vi "Make_SQL_for_basic_param.vi"(6 "Material Type":string, 8 "Porosity, %":string, 9 "Hardness HV, kg/mm2":string, 10 "Thickness, um":string, 11 "Breakdown DC voltage, V":string) -> (3 "result string":string)   [LabVIEW 2020]
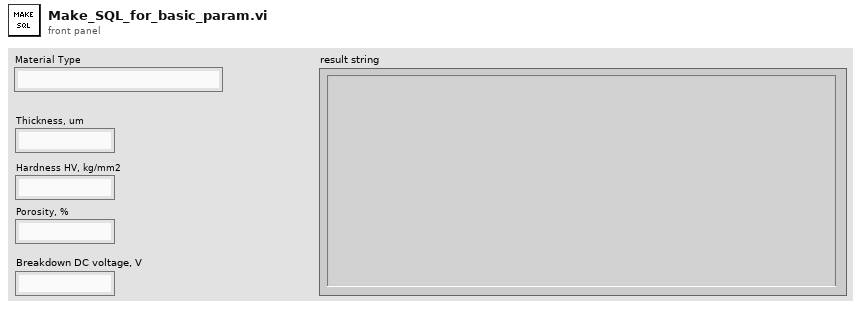
[diagram p1: front panel]
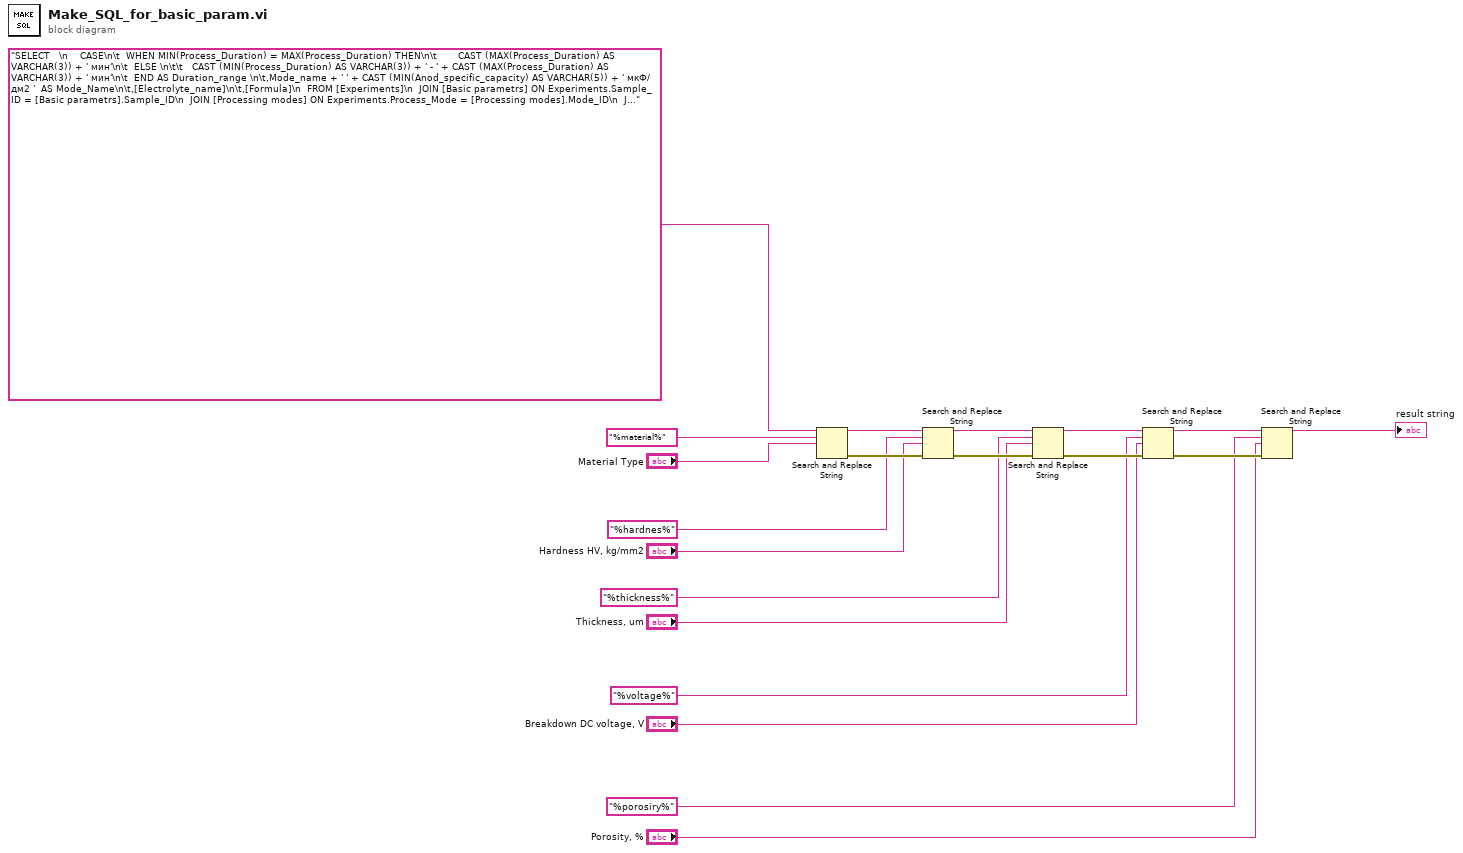
[diagram p0: block diagram]
diagram:
  n1 = Search and Replace String(input string="SELECT   \n    CASE\n\t  WHEN MIN(Process_Duration) = MAX(Process_Duration) THEN\n\t       CAST (MAX(Process_Duration) AS VARCHAR(3)) + ' мин'\n\t  ELSE \n\t\t   CAST (MIN(Process_Duration) AS VARCHAR(3)) + ' - ' + CAST (MAX(Process_Duration) AS VARCHAR(3)) + ' мин'\n\t  END AS Duration_range \n\t,Mode_name + ' ' + CAST (MIN(Anod_specific_capacity) AS VARCHAR(5)) + ' мкФ/дм2 '  AS Mode_Name\n\t,[Electrolyte_name]\n\t,[Formula]\n  FROM [Experiments]\n  JOIN [Basic parametrs] ON Experiments.Sample_ID = [Basic parametrs].Sample_ID\n  JOIN [Processing modes] ON Experiments.Process_Mode = [Processing modes].Mode_ID\n  JOIN [Materials] ON Experiments.Material = Materials.Material_ID\n  JOIN [Electrolytes] ON Experiments.Electrolyte = Electrolytes.Electrolyte_ID\n  WHERE Materials.[Type] = '%material%'  \n  AND [Basic parametrs].Hardnes_HV  %hardnes%\n  AND [Basic parametrs].Thickness_um  %thickness%\n  AND [Basic parametrs].Porosity  %porosiry%\n  AND [Basic parametrs].Breakdown_voltage_DC  %voltage%\n\n  GROUP BY Mode_name, Electrolyte_name, Formula\n", search string="%material%", replace string="Material Type") -> (result string=w15:string, error out=w19:errorcluster)  [unwired: 5 in, 2 out]
  n2 = Search and Replace String(input string=w15, search string="%hardnes%", replace string="Hardness HV, kg/mm2", error in=w19) -> (result string=w18:string, error out=w20:errorcluster)  [unwired: 4 in, 2 out]
  n3 = Search and Replace String(input string=w18, search string="%thickness%", replace string="Thickness, um", error in=w20) -> (result string=w10:string, error out=w11:errorcluster)  [unwired: 4 in, 2 out]
  n4 = Search and Replace String(input string=w10, search string="%voltage%", replace string="Breakdown DC voltage, V", error in=w11) -> (result string=w8:string, error out=w9:errorcluster)  [unwired: 4 in, 2 out]
  n5 = Search and Replace String(input string=w8, search string="%porosiry%", replace string="Porosity, %", error in=w9) -> (result string=→"result string":string)  [unwired: 4 in, 3 out]
